vi "E2_StatusSplit.vi"(11 "Input String":string) -> (3 "Output Cluster":T1)   [LabVIEW 2019, in "Instrument.Element2.lvclass"]
uses:
  Instrument.Element2.lvclass
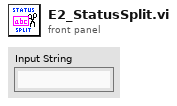
[diagram p1: front panel]
types:
  T1 = cluster{"Firmware":string, "[1]":string, "Serial No.":string, "[3]":string, "Laser Hrs.":string, "Year (YYYY)":string, "Month (MM)":string, "Date (DD)":string, "Hours (hh)":string, "Minutes (mm)":string, "Seconds (ss)":string, "[11]":string, "[12]":string, "Laser Status":string, "[14]":string, "Pump Status":string, "[16]":string, "[17]":string, "[18]":string, "[19]":string, "[20]":string, "[21]":string, "[22]":string, "[23]":string, "[24]":string, "[25]":string, "[26]":string, "Pico Speed":string, "Pico #":string, "[29]":string, "[30]":string, "[31]":string, "[32]":string, "[33]":string, "[34]":string, "[35]":string, "[36]":string, "[37]":string, "[38]":string, "[39]":string, "[40]":string, "[41]":string, "[42]":string, "[43]":string, "[44]":string, "[45]":string, "[46]":string, "[47]":string, "[48]":string, "[49]":string, "[50]":string, "[51]":string, "[52]":string, "[53]":string, "[54]":string, "[55]":string, "[56]":string, "[57]":string, "[58]":string, "[59]":string, "[60]":string, "[61]":string, "[62]":string, "[63]":string, "[64]":string, "[65]":string, "[66]":string, "[67]":string, "[68]":string, "[69]":string, "[70]":string, "[71]":string, "[72]":string, "[73]":string, "[74]":string, "Pump Laser 1":string, "Pump Laser 2":string, "Pump Laser 3":string, "Pump Laser 4":string, "Pump Laser 5":string, "[80]":string, "[81]":string, "[82]":string, "[83]":string, "[84]":string, "Diode Current Set":string, "Diode Current Actual":string, "[87]":string, "Power":string, "[89]":string, "[90]":string, "[91]":string, "Temp: Pump Chassis":string, "Temp: Pump Diodes":string, "Temp: Pump Tower":string, "Temp: Pump PCB":string, "SHG Point":string, "[97]":string, "[98]":string, "[99]":string, "[100]":string, "[101]":string, "[102]":string, "Spectrometer: Int. time":string, "[104]":string, "[105]":string, "[106]":string, "Starter: Duration":string, "Starter: Voltage":string, "Starter: PWM Mode":string, "Starter: Duty Cycle":string, "PowSensCtrlLoop: Kp":string, "PowSensCtrlLoop: Ki":string, "Cycle Time":string, "Max Pump Current":string, "Loop Status":string, "CrysPos: Move Interval":string, "CrysPos: Pico Steps":string, "CrysPos: Step Direction":string, "CrysPos: Max Moves":string, "CrysPos: Last Move":string, "CrysPos: Moves Done":string, "Temp: Control Unit":string, "Temp: Laser Head Pos 1":string, "Temp: Laser Head Pos 2":string, "[125]":string, "[126]":string, "[127]":string, "[128]":string, "[129]":string, "[130]":string, "[131]":string, "[132]":string, "[133]":string, "[134]":string, "[135]":string, "[136]":string, "[137]":string, "[138]":string, "[139]":string, "[140]":string, "[141]":string, "Wedge Control Counter":string, "[143]":string}
  T2 = cluster{"string array[0]":string, "string array[1]":string, "string array[2]":string, "string array[3]":string, "string array[4]":string, "string array[5]":string, "string array[6]":string, "string array[7]":string, "string array[8]":string, "string array[9]":string, "string array[10]":string, "string array[11]":string, "string array[12]":string, "string array[13]":string, "string array[14]":string, "string array[15]":string, "string array[16]":string, "string array[17]":string, "string array[18]":string, "string array[19]":string, "string array[20]":string, "string array[21]":string, "string array[22]":string, "string array[23]":string, "string array[24]":string, "string array[25]":string, "string array[26]":string, "string array[27]":string, "string array[28]":string, "string array[29]":string, "string array[30]":string, "string array[31]":string, "string array[32]":string, "string array[33]":string, "string array[34]":string, "string array[35]":string, "string array[36]":string, "string array[37]":string, "string array[38]":string, "string array[39]":string, "string array[40]":string, "string array[41]":string, "string array[42]":string, "string array[43]":string, "string array[44]":string, "string array[45]":string, "string array[46]":string, "string array[47]":string, "string array[48]":string, "string array[49]":string, "string array[50]":string, "string array[51]":string, "string array[52]":string, "string array[53]":string, "string array[54]":string, "string array[55]":string, "string array[56]":string, "string array[57]":string, "string array[58]":string, "string array[59]":string, "string array[60]":string, "string array[61]":string, "string array[62]":string, "string array[63]":string, "string array[64]":string, "string array[65]":string, "string array[66]":string, "string array[67]":string, "string array[68]":string, "string array[69]":string, "string array[70]":string, "string array[71]":string, "string array[72]":string, "string array[73]":string, "string array[74]":string, "string array[75]":string, "string array[76]":string, "string array[77]":string, "string array[78]":string, "string array[79]":string, "string array[80]":string, "string array[81]":string, "string array[82]":string, "string array[83]":string, "string array[84]":string, "string array[85]":string, "string array[86]":string, "string array[87]":string, "string array[88]":string, "string array[89]":string, "string array[90]":string, "string array[91]":string, "string array[92]":string, "string array[93]":string, "string array[94]":string, "string array[95]":string, "string array[96]":string, "string array[97]":string, "string array[98]":string, "string array[99]":string, "string array[100]":string, "string array[101]":string, "string array[102]":string, "string array[103]":string, "string array[104]":string, "string array[105]":string, "string array[106]":string, "string array[107]":string, "string array[108]":string, "string array[109]":string, "string array[110]":string, "string array[111]":string, "string array[112]":string, "string array[113]":string, "string array[114]":string, "string array[115]":string, "string array[116]":string, "string array[117]":string, "string array[118]":string, "string array[119]":string, "string array[120]":string, "string array[121]":string, "string array[122]":string, "string array[123]":string, "string array[124]":string, "string array[125]":string, "string array[126]":string, "string array[127]":string, "string array[128]":string, "string array[129]":string, "string array[130]":string, "string array[131]":string, "string array[132]":string, "string array[133]":string, "string array[134]":string, "string array[135]":string, "string array[136]":string, "string array[137]":string, "string array[138]":string, "string array[139]":string, "string array[140]":string, "string array[141]":string, "string array[142]":string, "string array[143]":string}
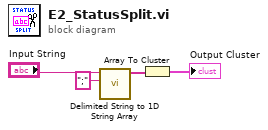
[diagram p0: block diagram]
diagram:
  n1 = call <vilib>:"Delimited String to 1D String Array.vi"("delimiter"=";", "delimited string"="Input String") -> ("string array"=w1:string[])  [unwired: 9 in]
  n2 = Array To Cluster(array=w1) -> (cluster=→"Output Cluster":T2)
